vi "input to tag bus.vi"(9 "indices":T1, 10 "data cluster":T2, 11 "tag bus in":T3) -> (3 "tag bus out":T3)   [LabVIEW 2017, in "RT Resource Usage runtime.lvclass"]
uses:
  RT Resource Usage runtime.lvclass
  <vilib>/NI/Tag Bus/table/data table.ctl
  input user data.ctl
  configuration/input data indices.ctl
  <vilib>/NI/Tag Bus/table/data polymorphs/write one/write Double.vi
  <vilib>/NI/Tag Bus/table/data polymorphs/write one/write Array of Double.vi
  <vilib>/NI/Tag Bus/table/data table.lvlib
  configuration/RT Resource Usage configuration.lvclass
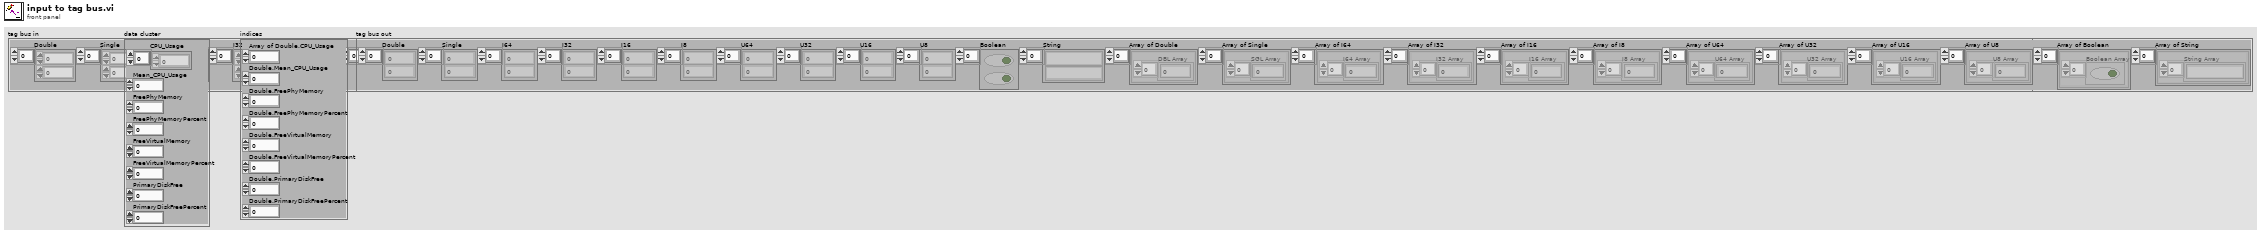
[diagram p1: front panel]
types:
  T1 = typedef "RT Resource Usage configuration.lvclass/input data indices.ctl" = cluster{"Array of Double.CPU_Usage":i32, "Double.Mean_CPU_Usage":i32, "Double.FreePhyMemory":i32, "Double.FreePhyMemoryPercent":i32, "Double.FreeVirtualMemory":i32, "Double.FreeVirtualMemoryPercent":i32, "Double.PrimaryDiskFree":i32, "Double.PrimaryDiskFreePercent":i32}
  T2 = typedef "RT Resource Usage runtime.lvclass/input user data.ctl" = cluster{"CPU_Usage":dbl[], "Mean_CPU_Usage":dbl, "FreePhyMemory":dbl, "FreePhyMemoryPercent":dbl, "FreeVirtualMemory":dbl, "FreeVirtualMemoryPercent":dbl, "PrimaryDiskFree":dbl, "PrimaryDiskFreePercent":dbl}
  T3 = typedef "tag bus.lvlib/data table.lvlib/data table.ctl" = cluster{"Double":dbl[], "Single":sgl[], "I64":i64[], "I32":i32[], "I16":i16[], "I8":i8[], "U64":u64[], "U32":u32[], "U16":u16[], "U8":u8[], "Boolean":bool[], "String":string[], "Array of Double":cluster{"DBL Array":dbl[]}[], "Array of Single":cluster{"SGL Array":sgl[]}[], "Array of I64":cluster{"I64 Array":i64[]}[], "Array of I32":cluster{"I32 Array":i32[]}[], "Array of I16":cluster{"I16 Array":i16[]}[], "Array of I8":cluster{"I8 Array":i8[]}[], "Array of U64":cluster{"U64 Array":u64[]}[], "Array of U32":cluster{"U32 Array":u32[]}[], "Array of U16":cluster{"U16 Array":u16[]}[], "Array of U8":cluster{"U8 Array":u8[]}[], "Array of Boolean":cluster{"Boolean Array":bool[]}[], "Array of String":cluster{"String Array":string[]}[]}
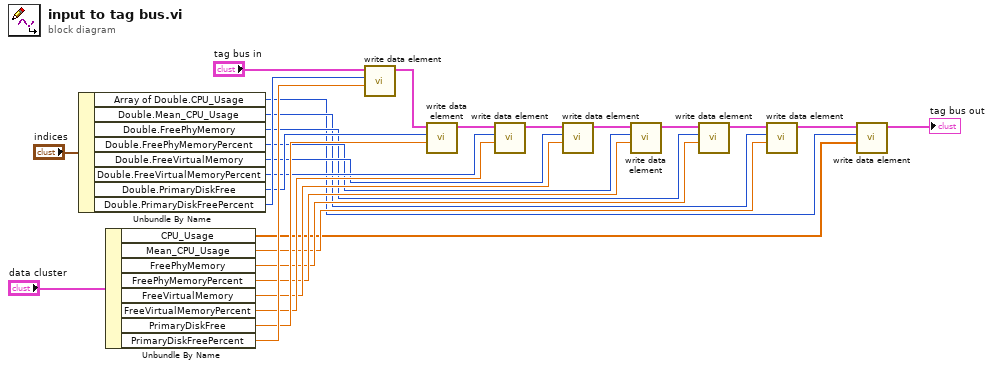
[diagram p0: block diagram]
diagram:
  n1 = Unbundle By Name("indices") -> ("Array of Double.CPU_Usage"=w4:i32, "Double.Mean_CPU_Usage"=w7:i32, "Double.FreePhyMemory"=w10:i32, "Double.FreePhyMemoryPercent"=w13:i32, "Double.FreeVirtualMemory"=w16:i32, "Double.FreeVirtualMemoryPercent"=w19:i32, "Double.PrimaryDiskFree"=w22:i32, "Double.PrimaryDiskFreePercent"=w25:i32)
  n2 = Unbundle By Name("data cluster") -> ("CPU_Usage"=w3:dbl[], "Mean_CPU_Usage"=w6:dbl, "FreePhyMemory"=w9:dbl, "FreePhyMemoryPercent"=w12:dbl, "FreeVirtualMemory"=w15:dbl, "FreeVirtualMemoryPercent"=w18:dbl, "PrimaryDiskFree"=w21:dbl, "PrimaryDiskFreePercent"=w24:dbl)
  n3 = call-poly <vilib>:"write data element.vi"("value"=w24, "index"=w25, "data table in"="tag bus in") -> ("data table out"=w20:T3)  [unwired: 8 in]
  n4 = call-poly <vilib>:"write data element.vi"("value"=w21, "index"=w22, "data table in"=w20) -> ("data table out"=w17:T3)  [unwired: 8 in]
  n5 = call-poly <vilib>:"write data element.vi"("value"=w18, "index"=w19, "data table in"=w17) -> ("data table out"=w14:T3)  [unwired: 8 in]
  n6 = call-poly <vilib>:"write data element.vi"("value"=w15, "index"=w16, "data table in"=w14) -> ("data table out"=w11:T3)  [unwired: 8 in]
  n7 = call-poly <vilib>:"write data element.vi"("value"=w12, "index"=w13, "data table in"=w11) -> ("data table out"=w8:T3)  [unwired: 8 in]
  n8 = call-poly <vilib>:"write data element.vi"("value"=w9, "index"=w10, "data table in"=w8) -> ("data table out"=w5:T3)  [unwired: 8 in]
  n9 = call-poly <vilib>:"write data element.vi"("value"=w6, "index"=w7, "data table in"=w5) -> ("data table out"=w2:T3)  [unwired: 8 in]
  n10 = call-poly <vilib>:"write data element.vi"("value"=w3, "index"=w4, "data table in"=w2) -> ("data table out"=→"tag bus out":T3)  [unwired: 8 in]
